vi "QMH API TESTER.vi"() -> ()   [LabVIEW 2019]
uses:
  User Events.lvlib
panel:
  in  "Start QMH":bool
  in  "stop":bool
  in  "Volts":dbl(knob) scale=0.0..10.0
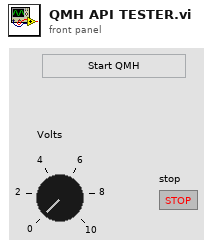
[diagram p1: front panel]
types:
  T1 = typedef "User Events.lvlib/User Events Typedef.ctl" = cluster{"Stop Event Interno":refnum<user-event>, "Volts":refnum<user-event>, "QMH Stop":refnum<user-event>, "Stop Event Externo":refnum<user-event>}
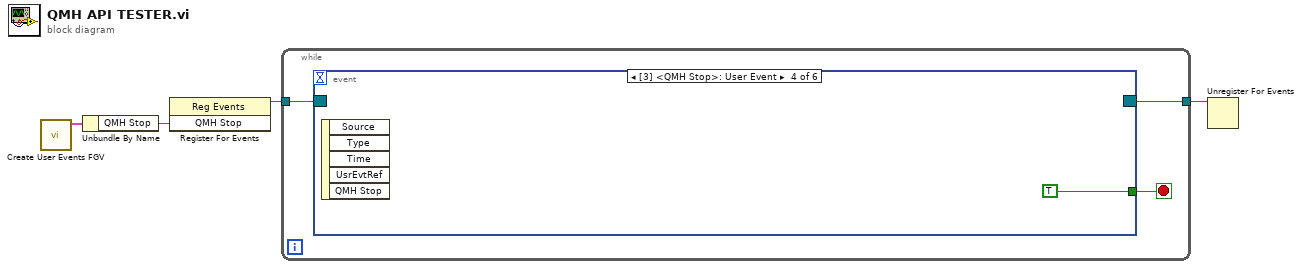
[diagram p0: block diagram]
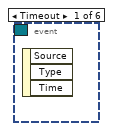
[diagram p2: hidden frame]
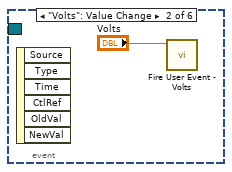
[diagram p3: hidden frame]
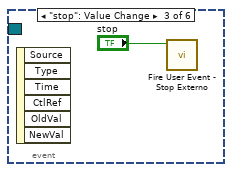
[diagram p4: hidden frame]
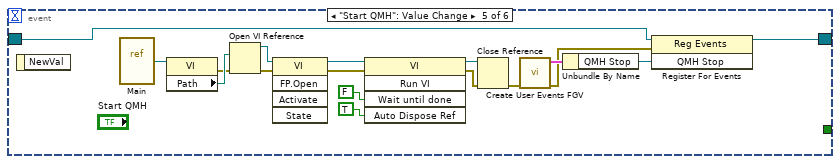
[diagram p5: hidden frame]
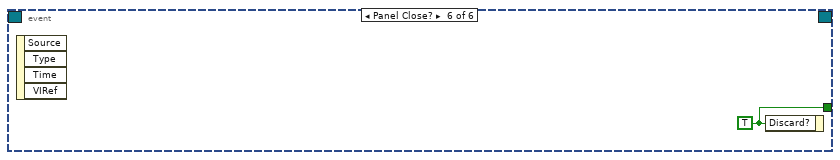
[diagram p6: hidden frame]
diagram:
  n1 = call "Create User Events FGV.vi"() -> ("User Events"=w3:T1)  [unwired: 10 in, 1 out]
  n2 = Unbundle By Name(w3) -> ("QMH Stop"=w2:refnum<user-event>)
  n3 = register-events(w2) -> (reference out=w4:refnum<event-registration>)  [unwired: 2 in, 1 out]
  n4 = while {
    tunnel: w4 -> [w6]
    tunnel: [w5] -> w1
    stop <- w7 stop-if-true
    n5 = event shown="[3] <QMH Stop>: User Event" {
      selector: w6 -> [_ _ _ _ w13 _]
      dyn-events: [_ _ _ _ w14 _] -> w5
      timeout: _ -> [_ _ _ _ _ _]
      tunnel: [_ _ _ TRUE ("Discard?") _ w28] -> w7
      event Timeout {
        n6 = event-data() -> ()  [unwired: 1 in, 3 out]
      }
      event "Volts": Value Change {
        n7 = event-data() -> ()  [unwired: 1 in, 6 out]
        n8 = call "Fire User Event - Volts.vi"("Volts"="Volts") -> ()  [unwired: 10 in, 1 out]
      }
      event "stop": Value Change {
        n9 = event-data() -> ()  [unwired: 1 in, 6 out]
        n10 = call "Fire User Event - Stop Externo.vi"("Stop Externo"="stop") -> ()  [unwired: 10 in, 1 out]
      }
      event User Event {
        n11 = event-data() -> ()  [unwired: 1 in, 5 out]
      }
      event "Start QMH": Value Change {
        n12 = event-data() -> ()  [unwired: 1 in, 1 out]
        n13 = vi-ref "Main.vi"() -> (w27:refnum<vi>)
        n14 = property class="VI"(reference=w27) -> (error out=w25:errorcluster, "Path"=w26:path)  [unwired: 1 in, 1 out]
        n15 = Open VI Reference(vi path=w26, error in (no error)=w25) -> (vi reference=w18:refnum<vi>, error out=w24:errorcluster)  [unwired: 4 in]
        n16 = invoke class="VI" method="FP.Open"(reference=w18, error in=w24) -> (reference out=w17:refnum<vi>, error out=w19:errorcluster)  [unwired: 3 in, 3 out]
        n17 = invoke class="VI" method="Run VI"(reference=w17, error in=w19, "Wait until done"=FALSE ("Wait Until Done"), "Auto Dispose Ref"=TRUE ("Auto Dispose Reference")) -> (reference out=w20:refnum<vi>, error out=w21:errorcluster)  [unwired: 1 in, 3 out]
        n18 = Close Reference(reference=w20, error in (no error)=w21) -> (error out=w12:errorcluster)
        n19 = call "Create User Events FGV.vi"("error in"=w12) -> ("error out"=w11:errorcluster, "User Events"=w15:T1)  [unwired: 9 in]
        n20 = Unbundle By Name(w15) -> ("QMH Stop"=w16:refnum<user-event>)
        n21 = register-events(reference=w13, error in=w11, w16) -> (reference out=w14:refnum<event-registration>)  [unwired: 1 out]
      }
      event Panel Close? {
        w28 = TRUE ("Discard?")
        n22 = event-data() -> ()  [unwired: 1 in, 4 out]
        n23 = event-data("Discard?"=w28) -> ()  [unwired: 1 in, 1 out]
      }
    }
  }
  n24 = Unregister For Events(event registration refnum=w1) -> ()  [unwired: 1 in, 1 out]
